vi "Set Speed.vi"(8 "error in":errorcluster, 10 "Pump %":dbl, 11 "Masterflex 75211 Settings":T1) -> (0 "error out":errorcluster, 1 "Connection Error":bool, 3 "Masterflex 75211 Settings 2":T1)   [LabVIEW 2018, in "Masterflex 75211.lvlib"]
uses:
  Masterflex 75211.lvlib
  Masterflex 75211 DAQ Setting.ctl
  <vilib>/DAQmx/write.llb/DAQmx Write (Analog DBL 1Chan 1Samp).vi
  <vilib>/DAQmx/write.llb/DAQmx Write (Digital Bool 1Line 1Point).vi
  <vilib>/DAQmx/miscellaneous.llb/DAQmx Fill In Error Info.vi
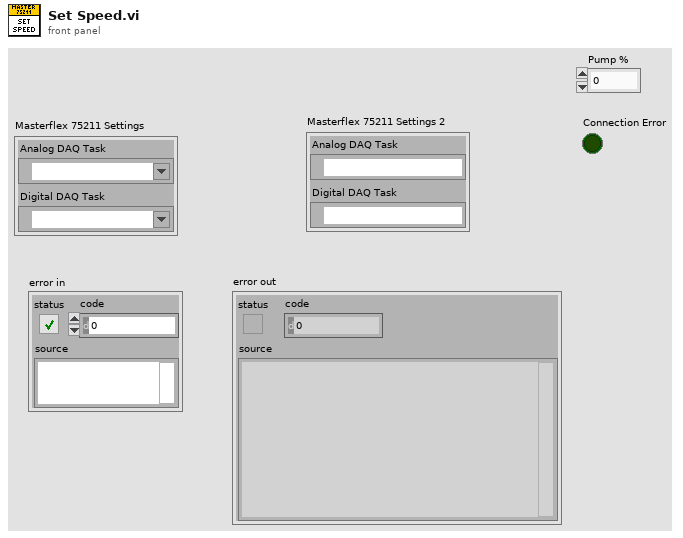
[diagram p1: front panel]
types:
  T1 = typedef "Masterflex 75211.lvlib/Masterflex 75211 DAQ Setting.ctl" = cluster{"Analog DAQ Task":refnum<k21>, "Digital DAQ Task":refnum<k21>}
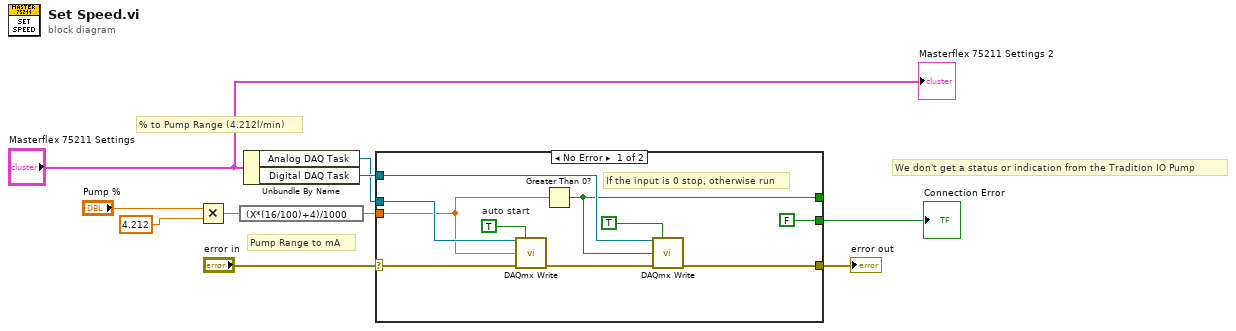
[diagram p0: block diagram]
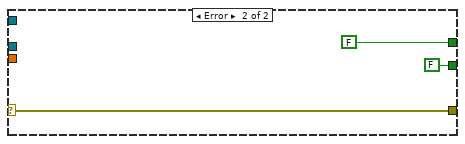
[diagram p2: hidden frame]
diagram:
  # "We don't get a status or indication from the Tradition IO Pump"
  # "% to Pump Range (4.212l/min)"
  # "Pump Range to mA"
  n1 = Multiply(x="Pump %", y=4.212 ("x")) -> (x*y=w4:dbl)
  n2 = expression code="(X*(16/100)+4)/1000"(w4) -> (w10:dbl)
  n3 = Unbundle By Name("Masterflex 75211 Settings") -> ("Analog DAQ Task"=w7:refnum<k21>, "Digital DAQ Task"=w8:refnum<k21>)
  n4 = case shown="No Error" "error in" {
    selector: "error in" -> [w12 w22]
    tunnel: w8 -> [w20 _]
    tunnel: w10 -> [w13 _]
    tunnel: w7 -> [w19 _]
    tunnel: [w14 w22] -> w6
    tunnel: [w16 FALSE ("Pump On?")] -> _
    tunnel: [FALSE ("Connection Error") FALSE ("Connection Error")] -> w3
    frame No Error {
      w17 = TRUE  # auto start
      # "If the input is 0 stop, otherwise run"
      n5 = call-poly <vilib>:"DAQmx Write.vi"("task/channels in"=w19, "auto start"=w17, "data"=w13, "error in"=w12) -> ("error out"=w15:errorcluster)  [unwired: 9 in, 2 out]
      n6 = Greater Than 0?(x=w13) -> (x > 0?=w16:bool)
      n7 = call-poly <vilib>:"DAQmx Write.vi"("task/channels in"=w20, "auto start"=TRUE, "data"=w16, "error in"=w15) -> ("error out"=w14:errorcluster)  [unwired: 9 in, 2 out]
    }
    frame Error {
    }
  }
  "error out" <- w6
  "Connection Error" <- w3
  "Masterflex 75211 Settings 2" <- "Masterflex 75211 Settings"
